vi "Delay Cycles set.vi"(6 "Infinite loop?":bool, 7 "Channel  (1: CH1)":u16(ring)=1 items=["CH1"=1, "CH2"=2, "CH3"=3, "CH4"=4], 8 "error in (no error)":errorcluster, 10 "Cycles(1~99999)":u32=1 min=1 max=99999, 11 "VISA resource name":refnum<visa-resource-name>) -> (0 "error out":errorcluster, 3 "VISA resource name out":refnum<visa-resource-name>)   [LabVIEW 2020, in "GPP.lvlib"]
uses:
  GPP.lvlib
  Function/VISA_COMMON.ctl
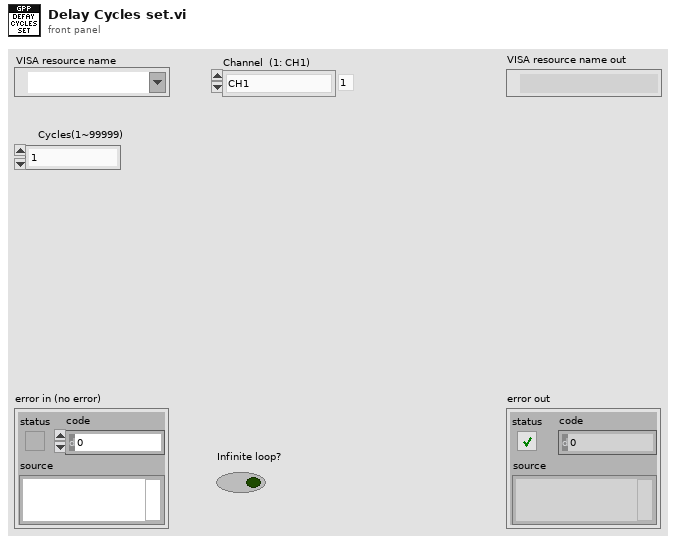
[diagram p1: front panel]
types:
  T1 = typedef "GPP.lvlib/VISA_COMMON.ctl" = enum16{"Initial", "Write CMD", "Read Result", "Read History", "Close"}
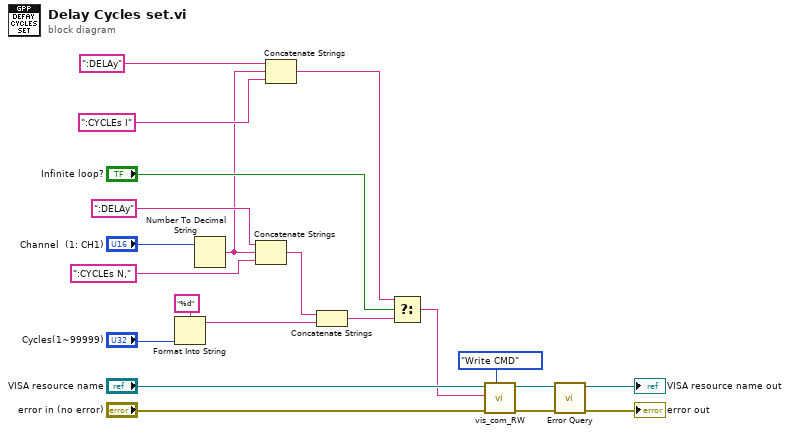
[diagram p0: block diagram]
diagram:
  n1 = Format Into String(format string="%d", "Cycles(1~99999)") -> (resulting string=w15:string)  [unwired: 2 in, 1 out]
  n2 = Number To Decimal String(number="Channel  (1: CH1)") -> (decimal integer string=w3:string)  [unwired: 1 in]
  n3 = Concatenate Strings(":DELAy", w3, ":CYCLEs N,") -> (w14:string)
  n4 = Concatenate Strings(":DELAy", w3, ":CYCLEs I") -> (w2:string)
  n5 = Concatenate Strings(w14, w15) -> (w8:string)
  n6 = Select(t=w2, s="Infinite loop?", f=w8) -> (s? t:f=w6:string)
  n7 = call "vis_com_RW.vi"("Funciton"=VISA_COMMON."Write CMD", "error in (no error)"="error in (no error)", "CMD String"=w6, "VISA resource in"="VISA resource name") -> ("error out"=w19:errorcluster, "VISA resource out"=w20:refnum<visa-resource-name>)  [unwired: 5 in, 1 out]
  n8 = call "Error Query.vi"("error in (no error)"=w19, "VISA resource name"=w20) -> ("error out"=→"error out":errorcluster, "VISA resource name out"=→"VISA resource name out":refnum<visa-resource-name>)  [unwired: 6 in, 2 out]
